vi "Get Inputs.vi"(8 "error in":errorcluster, 11 "CRDS in":refnum<class "CRDS.lvclass">) -> (0 "error out":errorcluster, 2 "Restart?":bool, 3 "CRDS out":refnum<class "CRDS.lvclass">)   [LabVIEW 2011, in "CRDS.lvclass"]
uses:
  CRDS.lvclass
  Program Files (x86)/National Instruments/LabVIEW 2011/resource/objmgr/daqmx.rc
  <vilib>/DAQmx/read.llb/DAQmx Read (Analog 2D I16 NChan NSamp).vi
  Data Class/Main Class/CRDS Data.lvclass
  Data Class/Cell Class/CRDS Cell Data.lvclass
  Reusable/Serial IO/Base/Serial IO.lvclass
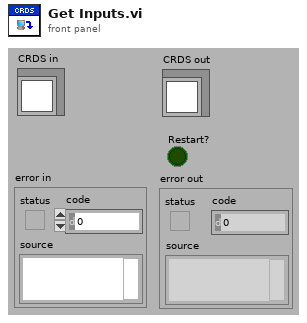
[diagram p1: front panel]
types:
  T1 = cluster{"YAG Ctr":refnum<k21>, "Diode Ctr":refnum<k21>, "Gated Ctr":refnum<k21>, "LF AI":refnum<k21>, "HF AI":refnum<k21>, "valveIn":refnum<k21>, "valveOut":refnum<k21>}
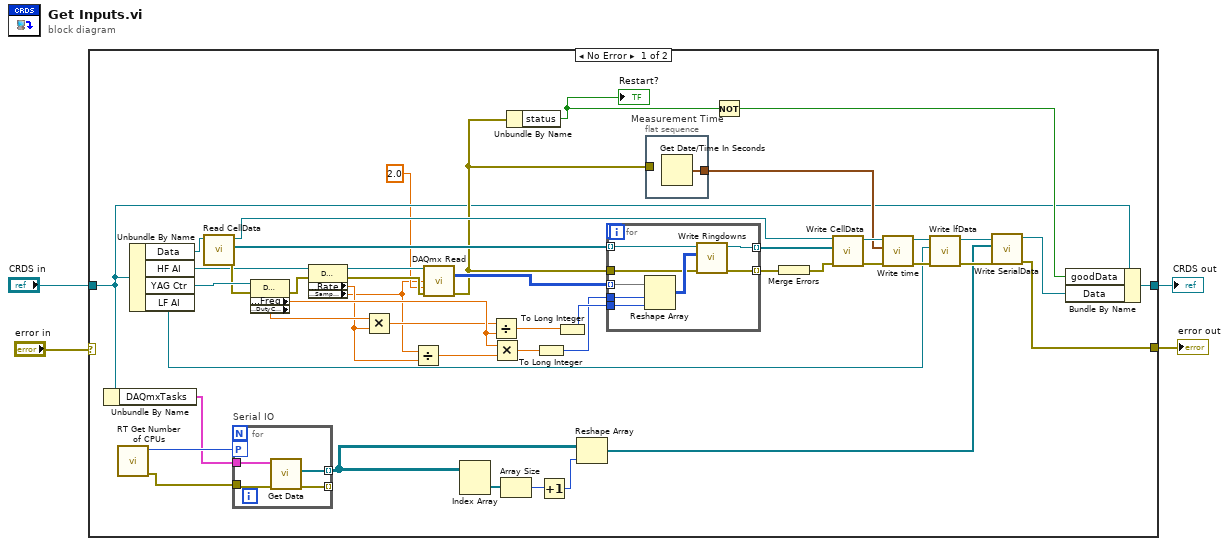
[diagram p0: block diagram]
diagram:
  n1 = case shown="No Error" "error in" {
    selector: "error in" -> [_ w65]
    tunnel: [w27 w66] -> w2
    tunnel: "CRDS in" -> [w14 w66]
    tunnel: [w15 w65] -> w1
    frame No Error {
      n2 = Unbundle By Name(w14) -> ("DAQmxTasks"=w13:T1)
      n3 = call <vilib>:"RT Get Number of CPUs.vi"() -> ("error out"=w20:errorcluster, "# of CPUs"=w24:u32)  [unwired: 10 in]
      n4 = Unbundle By Name(w14) -> ("Data"=w12:refnum<class "CRDS Data.lvclass">, "HF AI"=w10:refnum<k21>, "YAG Ctr"=w43:refnum<k21>, "LF AI"=w8:refnum<k21>)
      n5 = call "Read CellData.vi"("CRDS Data in"=w12) -> ("error out"=w30:errorcluster, "CellData"=w37:refnum<class "CRDS Cell Data.lvclass">[], "CRDS Data out"=w40:refnum<class "CRDS Data.lvclass">)  [unwired: 8 in]
      n6 = for "Serial IO" {
        tunnel: w13 -> [w55]
        workers-P: w24 -> [_]
        tunnel: [w54] -> w21 mode=indexing
        tunnel: w20 -> [w53]
        tunnel: [w52] -> _ mode=indexing
        n7 = call-dynamic "Get Data.vi"("error in (no error)"=w53, "Serial IO in"=w55) -> ("error out"=w52:errorcluster, "DataArray"=w54:refnum<class "Data.lvclass">[])  [unwired: 7 in, 1 out]
      }
      n8 = property class="DAQmx Channel"(reference=w43, error in=w30) -> (error out=w29:errorcluster, "CO.Pulse.Freq"=w50:dbl, "CO.Pulse.DutyCyc"=w51:dbl)  [unwired: 1 out]
      n9 = property class="DAQmx Timing"(reference=w10, error in=w29) -> (reference out=w31:refnum<k21>, error out=w28:errorcluster, "SampClk.Rate"=w42:dbl, "SampQuant.SampPerChan"=w9:dbl)
      n10 = Multiply(x=w51, y=w42) -> (x*y=w49:dbl)
      n11 = Divide(x=w9, y=w42) -> (x/y=w41:dbl)
      n12 = call-poly <vilib>:"DAQmx Read.vi"("task/channels in"=w31, "number of samples per channel"=w9, "timeout"=2.0, "error in"=w28) -> ("data"=w48:i16[][], "error out"=w35:errorcluster)  [unwired: 10 out]
      n13 = Index Array(array=w21) -> (element=w22:refnum<class "Data.lvclass">[])  [unwired: 2 in]
      n14 = Divide(x=w49, y=w50) -> (x/y=w46:dbl)
      n15 = Multiply(x=w50, y=w41) -> (x*y=w45:dbl)
      n16 = Array Size(array=w22) -> (size(s)=w6:i32)
      n17 = Unbundle By Name(w35) -> ("status"=w26:bool)
      "Restart?" <- w26
      n18 = To Long Integer(number=w45) -> (32bit integer=w44:i32)
      n19 = Increment(x=w6) -> (x+1=w5:i32)
      n20 = To Long Integer(number=w46) -> (32bit integer=w47:i32)
      n21 = Reshape Array(w21, w5) -> (w7:refnum<class "Data.lvclass">[])
      n22 = for {
        tunnel: w48 -> [w57] mode=indexing
        tunnel: w44 -> [w63]
        tunnel: w47 -> [w64]
        tunnel: w37 -> [w61] mode=indexing
        tunnel: [w60] -> w36 mode=indexing
        tunnel: w35 -> [w59]
        tunnel: [w58] -> w34 mode=indexing
        n23 = Reshape Array(w57, w63, w64) -> (w62:i16[][])
        n24 = call "Write Ringdowns.vi"("error in"=w59, "Ringdowns"=w62, "CRDS Cell Data in"=w61) -> ("error out"=w58:errorcluster, "CRDS Cell Data out"=w60:refnum<class "CRDS Cell Data.lvclass">)  [unwired: 7 in]
      }
      n25 = flat-sequence "Measurement Time" {
        tunnel: [w56] -> w38
        tunnel: w35 -> [_]
        frame #0 {
          n26 = Get Date/Time In Seconds() -> (seconds since 1Jan1904=w56:timestamp)
        }
      }
      n27 = Not(x=w26) -> (.not. x?=w25:bool)
      n28 = Merge Errors(w34) -> (w33:errorcluster)
      n29 = call "Write CellData.vi"("error in"=w33, "CellData"=w36, "CRDS Data in"=w40) -> ("error out"=w32:errorcluster, "CRDS Data out"=w39:refnum<class "CRDS Data.lvclass">)  [unwired: 7 in]
      n30 = call "Write time.vi"("error in (no error)"=w32, "time"=w38, "CRDS Data in"=w39) -> ("error out"=w18:errorcluster, "CRDS Data out"=w19:refnum<class "CRDS Data.lvclass">)  [unwired: 7 in]
      n31 = call "Write lfData.vi"("error in"=w18, "LF Task"=w8, "CRDS Data in"=w19) -> ("error out"=w16:errorcluster, "CRDS Data out"=w17:refnum<class "CRDS Data.lvclass">)  [unwired: 7 in]
      n32 = call "Write SerialData.vi"("error in (no error)"=w16, "SerialData"=w7, "CRDS Data in"=w17) -> ("error out"=w15:errorcluster, "CRDS Data out"=w23:refnum<class "CRDS Data.lvclass">)  [unwired: 7 in]
      n33 = Bundle By Name(cluster=w14, "goodData"=w25, "Data"=w23) -> (w27:refnum<class "CRDS.lvclass">)
    }
    frame Error {
    }
  }
  "error out" <- w1
  "CRDS out" <- w2
